vi "EZ-Zone String.vi"() -> ()   [LabVIEW 2011]
panel:
  out "Dnet Input Strings":string[](array[string])
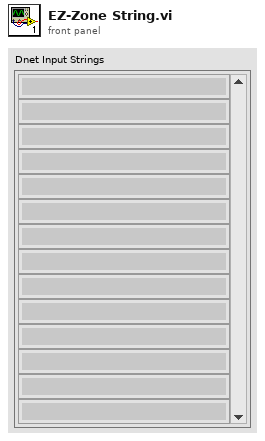
[diagram p1: front panel]
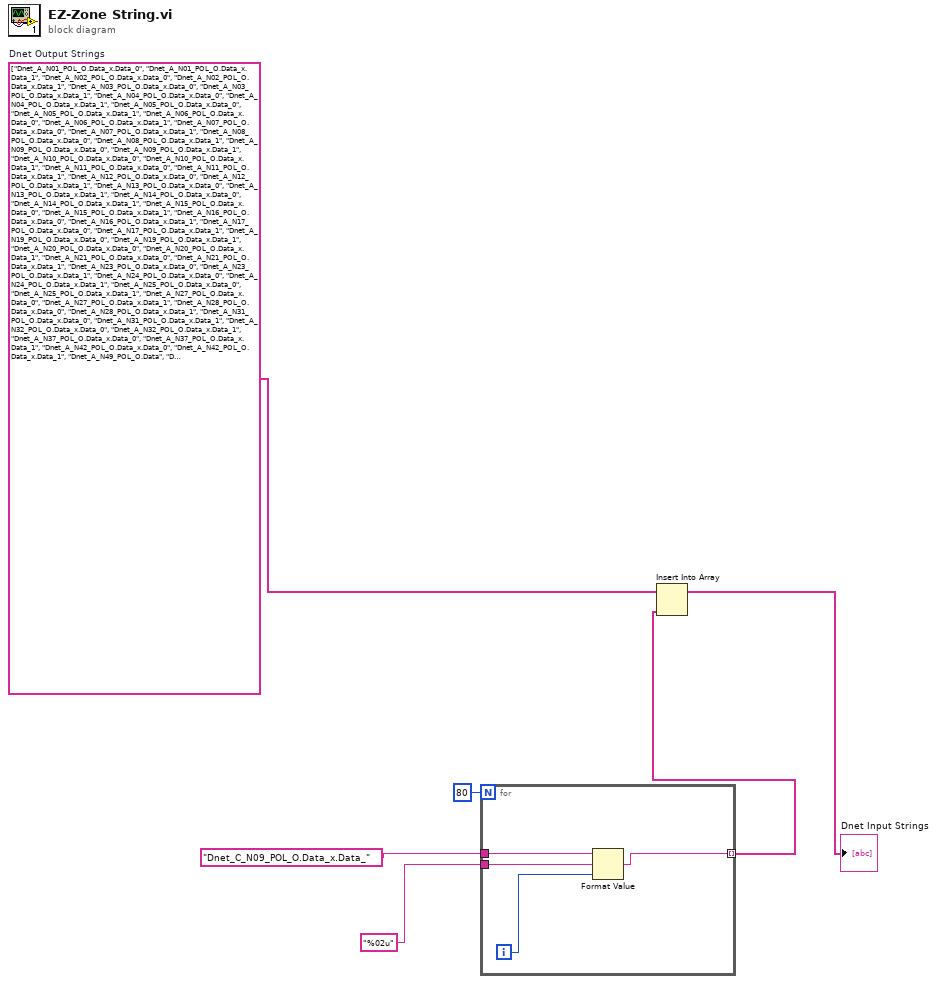
[diagram p0: block diagram]
diagram:
  w1 = string[] ["Dnet_A_N01_POL_O.Data_x.Data_0", "Dnet_A_N01_POL_O.Data_x.Data_1", "Dnet_A_N02_POL_O.Data_x.Data_0", "Dnet_A_N02_POL_O.Data_x.Data_1", "Dnet_A_N03_POL_O.Data_x.Data_0", "Dnet_A_N03_POL_O.Data_x.Data_1", "Dnet_A_N04_POL_O.Data_x.Data_0", "Dnet_A_N04_POL_O.Data_x.Data_1", "Dnet_A_N05_POL_O.Data_x.Data_0", "Dnet_A_N05_POL_O.Data_x.Data_1", "Dnet_A_N06_POL_O.Data_x.Data_0", "Dnet_A_N06_POL_O.Data_x.Data_1", "Dnet_A_N07_POL_O.Data_x.Data_0", "Dnet_A_N07_POL_O.Data_x.Data_1", "Dnet_A_N08_POL_O.Data_x.Data_0", "Dnet_A_N08_POL_O.Data_x.Data_1", "Dnet_A_N09_POL_O.Data_x.Data_0", "Dnet_A_N09_POL_O.Data_x.Data_1", "Dnet_A_N10_POL_O.Data_x.Data_0", "Dnet_A_N10_POL_O.Data_x.Data_1", "Dnet_A_N11_POL_O.Data_x.Data_0", "Dnet_A_N11_POL_O.Data_x.Data_1", "Dnet_A_N12_POL_O.Data_x.Data_0", "Dnet_A_N12_POL_O.Data_x.Data_1", "Dnet_A_N13_POL_O.Data_x.Data_0", "Dnet_A_N13_POL_O.Data_x.Data_1", "Dnet_A_N14_POL_O.Data_x.Data_0", "Dnet_A_N14_POL_O.Data_x.Data_1", "Dnet_A_N15_POL_O.Data_x.Data_0", "Dnet_A_N15_POL_O.Data_x.Data_1", "Dnet_A_N16_POL_O.Data_x.Data_0", "Dnet_A_N16_POL_O.Data_x.Data_1", "Dnet_A_N17_POL_O.Data_x.Data_0", "Dnet_A_N17_POL_O.Data_x.Data_1", "Dnet_A_N19_POL_O.Data_x.Data_0", "Dnet_A_N19_POL_O.Data_x.Data_1", "Dnet_A_N20_POL_O.Data_x.Data_0", "Dnet_A_N20_POL_O.Data_x.Data_1", "Dnet_A_N21_POL_O.Data_x.Data_0", "Dnet_A_N21_POL_O.Data_x.Data_1", "Dnet_A_N23_POL_O.Data_x.Data_0", "Dnet_A_N23_POL_O.Data_x.Data_1", "Dnet_A_N24_POL_O.Data_x.Data_0", "Dnet_A_N24_POL_O.Data_x.Data_1", "Dnet_A_N25_POL_O.Data_x.Data_0", "Dnet_A_N25_POL_O.Data_x.Data_1", "Dnet_A_N27_POL_O.Data_x.Data_0", "Dnet_A_N27_POL_O.Data_x.Data_1", "Dnet_A_N28_POL_O.Data_x.Data_0", "Dnet_A_N28_POL_O.Data_x.Data_1", "Dnet_A_N31_POL_O.Data_x.Data_0", "Dnet_A_N31_POL_O.Data_x.Data_1", "Dnet_A_N32_POL_O.Data_x.Data_0", "Dnet_A_N32_POL_O.Data_x.Data_1", "Dnet_A_N37_POL_O.Data_x.Data_0", "Dnet_A_N37_POL_O.Data_x.Data_1", "Dnet_A_N42_POL_O.Data_x.Data_0", "Dnet_A_N42_POL_O.Data_x.Data_1", "Dnet_A_N49_POL_O.Data", "Dnet_A_N49_POL_O.Data1", "Dnet_A_N49_POL_O.ExtendedData", "Dnet_A_N50_POL_O.Data_x.Data_0", "Dnet_A_N50_POL_O.Data_x.Data_1", "Dnet_A_N51_POL_O.Data_x.Data_0", "Dnet_A_N51_POL_O.Data_x.Data_1", "Dnet_A_N53_POL_O.Data", "Dnet_A_N53_POL_O.Data1", "Dnet_A_N53_POL_O.ExtendedData", "Dnet_A_N54_POL_O.Data", "Dnet_A_N54_POL_O.Data1", "Dnet_A_N54_POL_O.ExtendedData", "Dnet_A_N55_POL_O.Data_x.Data_0", "Dnet_A_N55_POL_O.Data_x.Data_1", "Dnet_A_N56_POL_O.Data_x.Data_0", "Dnet_A_N56_POL_O.Data_x.Data_1", "Dnet_B_N01_POL_O.Data_x.Data_0", "Dnet_B_N01_POL_O.Data_x.Data_1", "Dnet_B_N02_POL_O.Data_x.Data_0", "Dnet_B_N02_POL_O.Data_x.Data_1", "Dnet_B_N03_POL_O.Data_x.Data_0", "Dnet_B_N03_POL_O.Data_x.Data_1", "Dnet_B_N04_POL_O.Data_x.Data_0", "Dnet_B_N04_POL_O.Data_x.Data_1", "Dnet_B_N05_POL_O.Data_x.Data_0", "Dnet_B_N05_POL_O.Data_x.Data_1", "Dnet_B_N06_POL_O.Data_x.Data_0", "Dnet_B_N06_POL_O.Data_x.Data_1", "Dnet_B_N08_POL_O.Data_x.Data_0", "Dnet_B_N08_POL_O.Data_x.Data_1", "Dnet_B_N09_POL_O.Data_x.Data_0", "Dnet_B_N09_POL_O.Data_x.Data_1", "Dnet_B_N10_POL_O.Data_x.Data_0", "Dnet_B_N10_POL_O.Data_x.Data_1", "Dnet_B_N11_POL_O.Data_x.Data_0", "Dnet_B_N11_POL_O.Data_x.Data_1", "Dnet_B_N12_POL_O.Data_x.Data_0", "Dnet_B_N12_POL_O.Data_x.Data_1", "Dnet_B_N13_POL_O.Data_x.Data_0", "Dnet_B_N13_POL_O.Data_x.Data_1", "Dnet_B_N14_POL_O.Data_x.Data_0", "Dnet_B_N14_POL_O.Data_x.Data_1", "Dnet_B_N15_POL_O.Data_x.Data_0", "Dnet_B_N15_POL_O.Data_x.Data_1", "Dnet_B_N21_POL_O.Data", "Dnet_C_N01_POL_O.Data_x.Data_0", "Dnet_C_N01_POL_O.Data_x.Data_1", "Dnet_C_N02_POL_O.Data_x.Data_0", "Dnet_C_N02_POL_O.Data_x.Data_1", "Dnet_C_N03_POL_O.Data_x.Data_0", "Dnet_C_N03_POL_O.Data_x.Data_1", "Dnet_C_N04_POL_O.Data_x.Data_0", "Dnet_C_N04_POL_O.Data_x.Data_1", "Dnet_C_N05_POL_O.Data_x.Data_0", "Dnet_C_N05_POL_O.Data_x.Data_1", "Dnet_C_N06_POL_O.Data_x.Data_0", "Dnet_C_N06_POL_O.Data_x.Data_1", "Dnet_C_N07_POL_O.Data_x.Data_0", "Dnet_C_N07_POL_O.Data_x.Data_1", "Dnet_C_N08_POL_O.Data_x.Data_0", "Dnet_C_N08_POL_O.Data_x.Data_1"]  # Dnet Output Strings
  n1 = for {
    N: 80 -> [_]
    tunnel: "Dnet_C_N09_POL_O.Data_x.Data_" -> [w10]
    tunnel: "%02u" -> [w9]
    tunnel: [w7] -> w3 mode=indexing
    i -> [w8]
    n2 = Format Value(string ("")=w10, format string=w9, value (0)=w8) -> (output string=w7:string)
  }
  n3 = Insert Into Array(array=w1, new element=w3) -> (→"Dnet Input Strings":string[])  [unwired: 1 in]
